vi "Unregister Callbacks.vi"(8 "error in (no error)":errorcluster, 11 "Callbacks":T1) -> (0 "error out":errorcluster)   [LabVIEW 2020, in "NI_VS UI Tree Alias Browser.lvlib"]
uses:
  <vilib>/NI VeriStand/UI Controls/Tree and Alias Browser/NI_VS UI Tree Alias Browser.lvlib
  <vilib>/NI VeriStand/UI Controls/Tree and Alias Browser/Callback Type.ctl
  <vilib>/NI VeriStand/UI Controls/Tree and Alias Browser/Net Event Data Ref.ctl
  <vilib>/NI VeriStand/UI Controls/Tree and Alias Browser/Net Event Data.ctl
  <vilib>/NI VeriStand/UI Controls/Tree and Alias Browser/Net Event.ctl
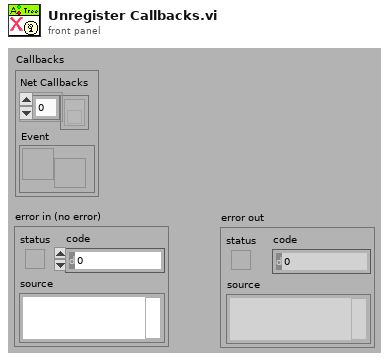
[diagram p1: front panel]
types:
  T1 = typedef "NI_VS UI Tree Alias Browser.lvlib/Callback Type.ctl" = cluster{"Net Callbacks":refnum<k27>[], "Event":T2}
  T2 = typedef "NI_VS UI Tree Alias Browser.lvlib/Net Event Data Ref.ctl" = refnum<user-event>
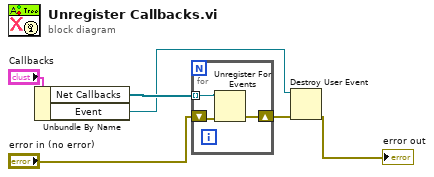
[diagram p0: block diagram]
diagram:
  n1 = Unbundle By Name("Callbacks") -> ("Net Callbacks"=w6:refnum<k27>[], "Event"=w5:T2)
  n2 = for {
    tunnel: w6 -> [w9] mode=indexing
    shift-right: [w7] -> w4
    shift-left: "error in (no error)" -> [w8]
    n3 = Unregister For Events(event registration refnum=w9, error in=w8) -> (error out=w7:errorcluster)
  }
  n4 = Destroy User Event(user event=w5, error in=w4) -> (error out=→"error out":errorcluster)
